vi "Read azError.vi"(8 "error in (no error)":errorcluster, 11 "AzElError in":refnum<class "AzElError.lvclass">) -> (0 "error out":errorcluster, 2 "azError":dbl[unit]=0.0001454441043328608, 3 "AzElError out":refnum<class "AzElError.lvclass">)   [LabVIEW 2022 SP3, in "TCSDataDefinitions.lvlib" / "TCSPublicStatus.lvlib" / "PointingPositions.lvlib" / "AzElError.lvclass"]
uses:
  AzElError.lvclass
  AzElError.lvclass/AzElError.ctl
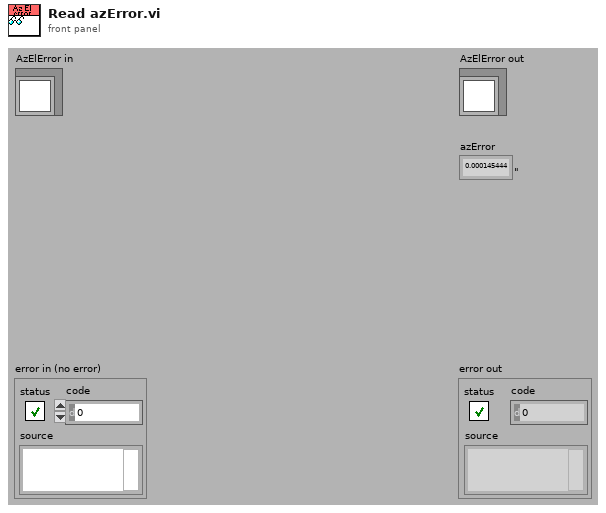
[diagram p1: front panel]
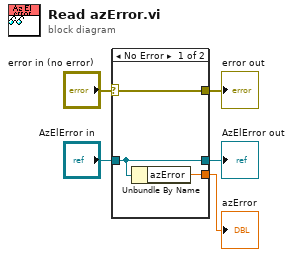
[diagram p0: block diagram]
diagram:
  n1 = case shown="No Error" "error in (no error)" {
    selector: "error in (no error)" -> [w8 w9]
    tunnel: [w8 w9] -> w4
    tunnel: [w7 w10] -> w2
    tunnel: "AzElError in" -> [w7 w10]
    tunnel: [w6 _] -> w1
    frame No Error {
      n2 = Unbundle By Name(w7) -> ("azError"=w6:dbl[unit])
    }
    frame Error {
    }
  }
  "error out" <- w4
  "AzElError out" <- w2
  "azError" <- w1
